vi "Write Actor Name.vi"(8 "error in (no error)":errorcluster, 10 "Actor Name":string, 11 "Generic Actor in":refnum<class "Generic Actor.lvclass">) -> (0 "error out":errorcluster, 3 "Generic Actor out":refnum<class "Generic Actor.lvclass">)   [LabVIEW 2020, in "Generic Actor.lvlib" / "Generic Actor.lvclass"]
uses:
  Generic Actor.lvclass
  Generic Actor.lvclass/Generic Actor.ctl
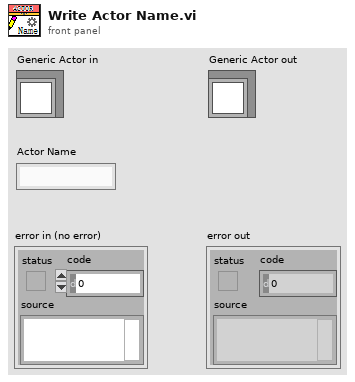
[diagram p1: front panel]
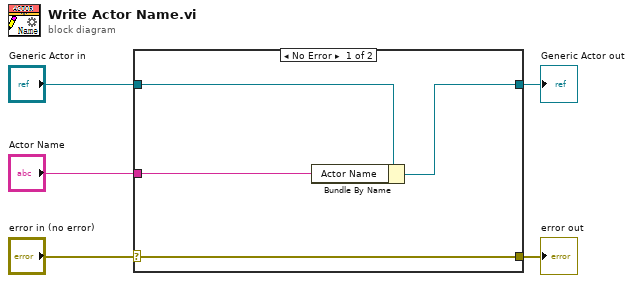
[diagram p0: block diagram]
diagram:
  n1 = case shown="No Error" "error in (no error)" {
    selector: "error in (no error)" -> [w9 w10]
    tunnel: [w9 w10] -> w4
    tunnel: [w7 w11] -> w2
    tunnel: "Generic Actor in" -> [w8 w11]
    tunnel: "Actor Name" -> [w6 _]
    frame No Error {
      n2 = Bundle By Name(cluster=w8, "Actor Name"=w6) -> (w7:refnum<class "Generic Actor.lvclass">)
    }
    frame Error {
    }
  }
  "error out" <- w4
  "Generic Actor out" <- w2
